vi "DisplayExecutionCallback.vi"(4 "User Parameter":T1, 5 "Event Data":cluster{"exec":refnum<k7>, "reason":i32}, 6 "Control Ref":refnum<k7>, 7 "Event Common Data":T2) -> ()   [LabVIEW 2010]
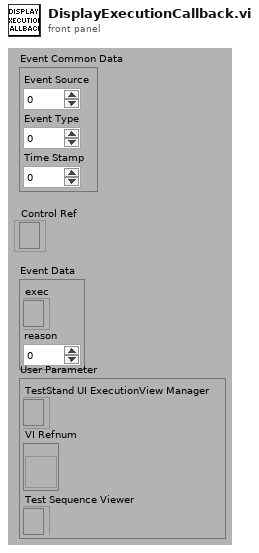
[diagram p1: front panel]
types:
  T1 = cluster{"TestStand UI ExecutionView Manager":refnum<k7>, "VI Refnum":refnum<vi>, "Test Sequence Viewer":refnum<k7>}
  T2 = cluster{"Event Source":i32, "Event Type":u32, "Time Stamp":u32}
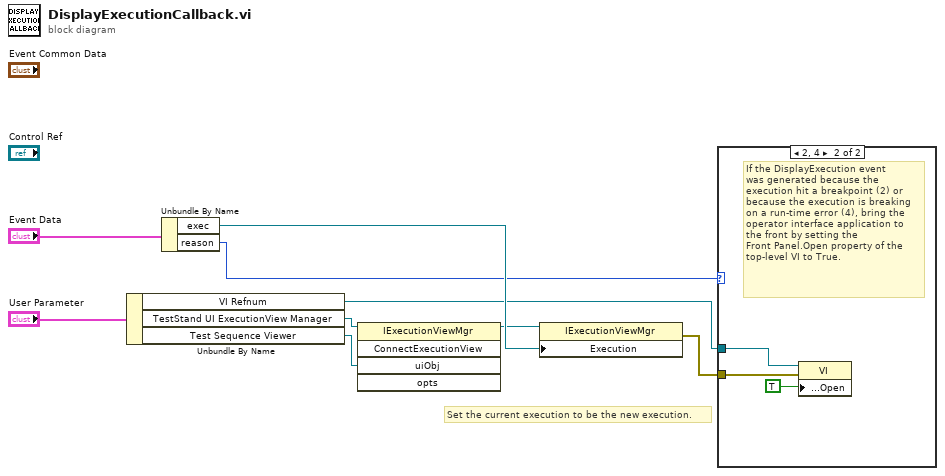
[diagram p0: block diagram]
diagram:
  # "Set the current execution to be the new execution."
  n1 = Unbundle By Name("User Parameter") -> ("VI Refnum"=w5:refnum<vi>, "TestStand UI ExecutionView Manager"=w6:refnum<k7>, "Test Sequence Viewer"=w1:refnum<k7>)
  n2 = Unbundle By Name("Event Data") -> ("exec"=w9:refnum<k7>, "reason"=w8:i32)
  n3 = invoke class="IExecutionViewMgr" method="ConnectExecutionView"(reference=w6, "uiObj"=w1) -> (reference out=w2:refnum<k7>)  [unwired: 3 in, 4 out]
  n4 = property class="IExecutionViewMgr"(reference=w2, "Execution"=w9) -> (error out=w7:errorcluster)  [unwired: 1 in, 1 out]
  n5 = case shown="2, 4" w8 {
    tunnel: w7 -> [_ w12]
    tunnel: w5 -> [_ w11]
    frame Default {
    }
    frame 2, 4 {
      # "If the DisplayExecution event\nwas generated because the\nexecution hit a breakpoint (2) or\nbecause the execution is breaking\non a run-time error (4), bring the\noperator interface application to\nthe front by setting the\nFront Panel.Open property of the\ntop-level VI to True."
      n6 = property class="VI"(reference=w11, error in=w12, "Front Panel Window:Open"=TRUE) -> ()  [unwired: 2 out]
    }
  }
